vi "target_old.vi"() -> ()   [LabVIEW 2011]
uses:
  Output - Cluster.ctl
  Input - Cluster.ctl
  <vilib>/Platform/TimedLoop/XDataNode/timing_clust.ctl
  <vilib>/Platform/TimedLoop/XDataNode/nitl_modes.ctl
  <vilib>/Platform/TimedLoop/XDataNode/wakeup.ctl
  <vilib>/functionblocks/Counter/Count Up/Count Up.vi
  <vilib>/functionblocks/Control/PID/PID.vi
  <vilib>/Platform/TimedLoop/XDataNode/XDataNode.xnode
  <vilib>/functionblocks/FB Core/FB Core.xnode
  <vilib>/Platform/TimedLoop/XDataNode/XDNodeRunTimeDep.lvlib
  <vilib>/functionblocks/NI_FunctionBlock Libraries.lvlib
panel:
  in  "Output - Cluster":T1 {"DS-3 [bar]" format="%#.2g"; "TS-6 [°C]" format="%#.2g"; "GZ-1 [dl]" format="%.0g"; "TS-5 [°C]" format="%#.2g"; "pHS-1 [pH]" format="%.2g"; "TS-4 [°C]" format="%#.2g"; "FS-2 [l]" format="%.2g"; "FS-1 [l]" format="%.2g"}
  # "The Network Variable Engine and Variable Client Support must be installed on the RT target\nfor this application to function properly. If the Network Variable Engine is not supported on\nthe target (e.g.  FP-2000 with <32MB of RAM), open the project and move the variable library\nto My Computer in the project. Doing this will deploy the variables to localhost but\nwill still require that Variable Client Support be installed on the RT target."
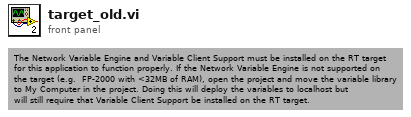
[diagram p1: front panel]
types:
  T1 = typedef "Output - Cluster.ctl" = cluster{"DFS-1 [dl]":u64, "FS-3 [l]":dbl, "DFS-1 [l/min]":dbl, "DS-1 [bar]":dbl, "V-10 ZU":bool, "V-14 ZU":bool, "FS-1 [l]":dbl, "FS-2 [l]":dbl, "TS-4 [°C]":dbl, "HS-1":bool, "V-13 [%]":u8, "V-15 [%]":u8, "P-4 [%]":u8, "P-5 [%]":u8, "Dosierung":bool, "MR Max Füllstand":bool, "MR Min Füllstand":bool, "Dosiermenge [l]":sgl, "V-14 AUF":bool, "V-10 AUF":bool, "T-1 Max Füllstand":bool, "T-1 Min Füllstand":bool, "T-2 Max Füllstand":bool, "T-2 Min Füllstand":bool, "pHS-1 [pH]":dbl, "P-4 RUN":bool, "P-5 RUN ":bool, "V-33 AUF":bool, "V-33 ZU":bool, "V-34 AUF":bool, "V-34 ZU":bool, "P-4 ERR":bool, "P-5 ERR":bool, "TS-5 [°C]":dbl, "GZ-1 [dl]":u64, "TS-6 [°C]":dbl, "DS-3 [bar]":dbl}
  T2 = cluster{"Durchflussregelung":dbl, "Temperaturregelung":bool, "STOP":bool, "Period":i64, "Zirkulation":u64, "Dosierung Zeit":u64}
  T3 = typedef "XDNodeRunTimeDep.lvlib/timing_clust.ctl" = cluster{"Expected End [f-1]":u64, "Actual End [f-1]":u64, "Finished Late? [f-1]":bool, "Expected End [i-1]":u64, "Actual End [i-1]":u64, "Finished Late? [i-1]":bool, "Expected Start [i]":u64, "Actual Start [i]":u64, "Expected Start [f]":u64, "Actual Start [f]":u64, "Source Name":string, "Structure Name":string, "Period":i64, "Deadline":i64, "Offset":i64, "Start":i64, "Priority":i32, "Timeout":i32, "Mode":T4, "Wakeup Reason":T5, "Error":errorcluster, "Source Type":string, "Secondary Source Type":string, "Global End Time":u64, "Global Start Time":u64, "Frame Duration":u64, "Iteration Duration":u64, "Assigned CPU":i32, "I/O Scan Engine Mode":u32}
  T4 = typedef "XDNodeRunTimeDep.lvlib/nitl_modes.ctl" = enum32{"No Change", "Process missed periods, maintain original phase", "Discard missed periods, maintain original phase", "Process missed periods, ignore original phase", "Discard missed periods, ignore original phase"}
  T5 = typedef "XDNodeRunTimeDep.lvlib/wakeup.ctl" = enum32{"Normal", "Aborted", "Asynchronous wakeup", "Timing source error", "Timed loop error", "Timeout"}
  T6 = enum16{"open", "replace", "create", "open or create", "replace or create", "replace or create with confirmation"}
  T7 = typedef "Input - Cluster.ctl" = cluster{"V-13 [%]":u8, "V-15 [%]":u8, "Log-Target":bool, "P-4":bool, "P-4 Drehzahl [%]":u8, "Temperaturregelung":bool, "Überdruckregelung":bool, "Füllstandsregulierung":bool, "V-10":bool, "Log-Host":bool, "V-14":bool, "P-5":bool, "P-5 Drehzahl [%]":u8, "HS-1":bool, "Füllstand  P":sgl, "Füllstand I":sgl, "Füllstand D":sgl, "Füllstand Soll [l]":sgl, "Druck  P":sgl, "Druck I":sgl, "Druck D":sgl, "Druck Soll [bar]":sgl, "Temp Soll [°C]":sgl, "Dosierung":bool, "Dosiermenge [l]":sgl, "Dosiergeschw. [l/min]":sgl, "Tank":bool, "Hysterese [°C]":sgl, "MR Füllstandsüberwachung":bool, "Tank Füllstandsüberwachung":bool, "Log Target [ms]":u32, "Log Host [s]":u32, "P-5 EIN [min]":u8, "P-5 AUS [min]":u8, "Zirkulation":bool, "V-33":bool, "V-34":bool}
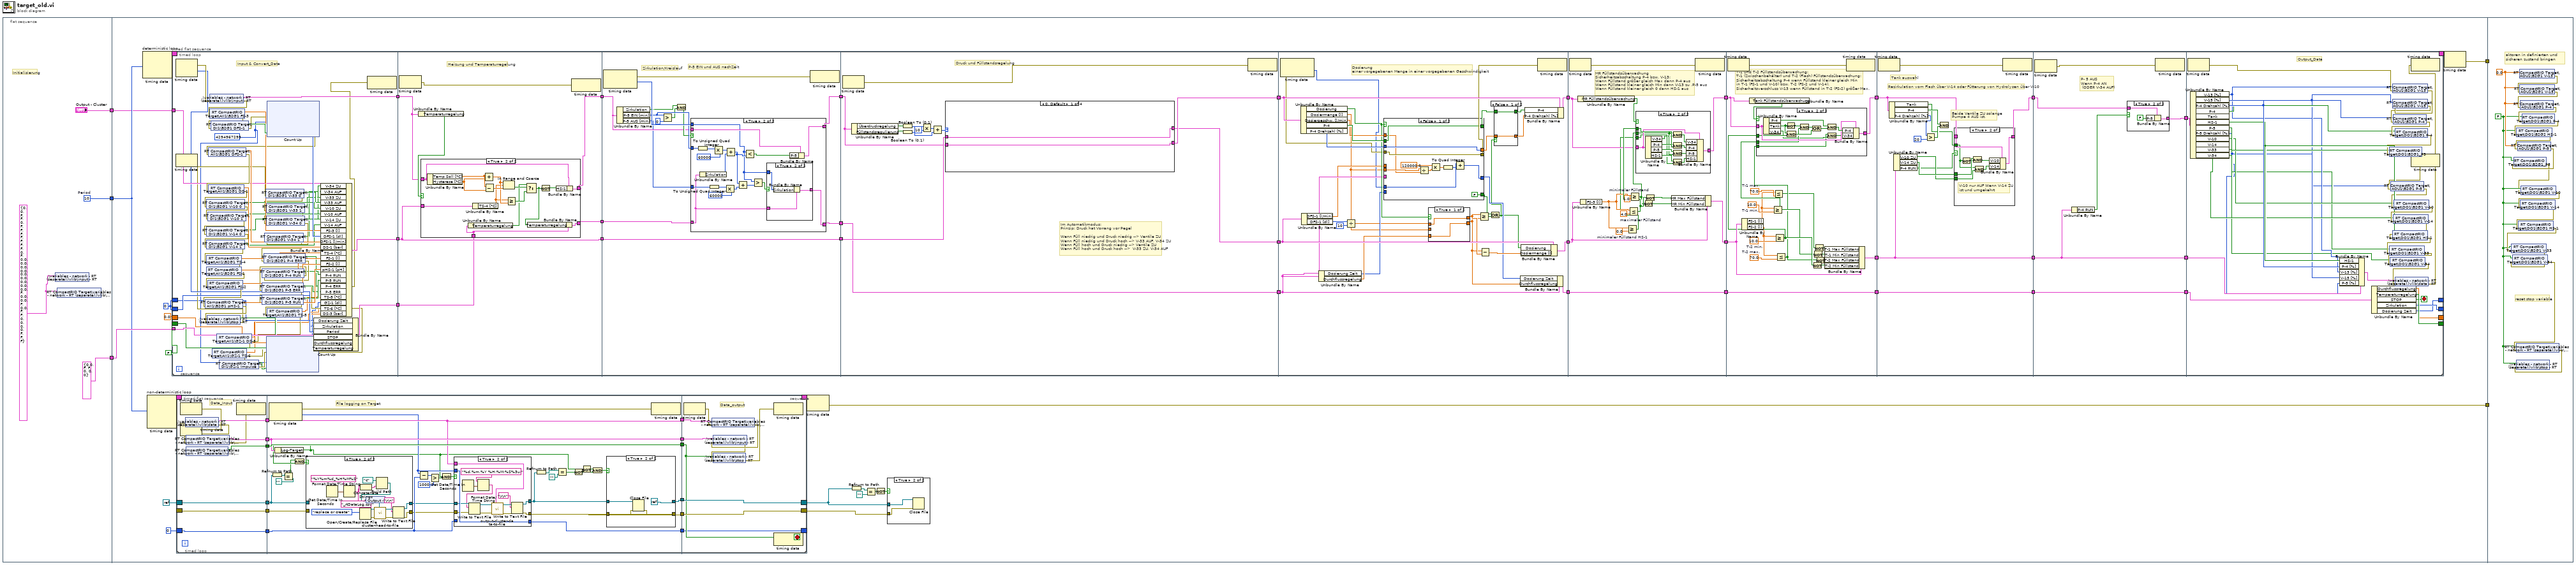
[diagram p0: block diagram]
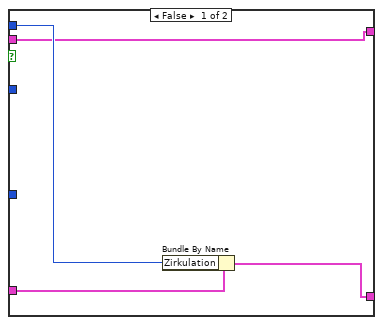
[diagram p7: hidden frame]
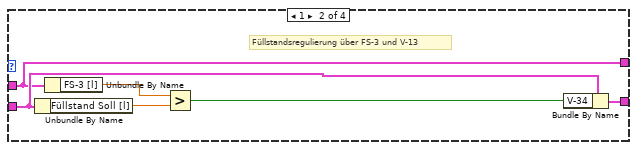
[diagram p9: hidden frame]
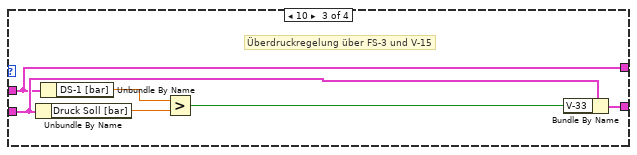
[diagram p10: hidden frame]
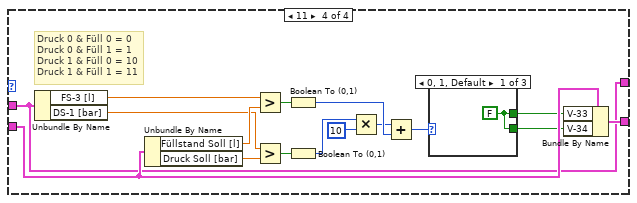
[diagram p11: hidden frame]
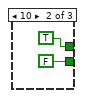
[diagram p12: hidden frame]
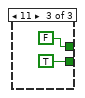
[diagram p13: hidden frame]
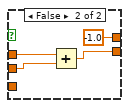
[diagram p14: hidden frame]
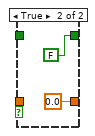
[diagram p15: hidden frame]
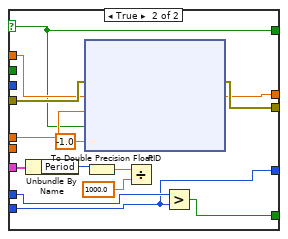
[diagram p16: hidden frame]
diagram:
  n1 = flat-sequence {
    tunnel: [T2 {"Durchflussregelung"=0.0, "Temperaturregelung"=FALSE, "STOP"=FALSE, "Period"=0, "Zirkulation"=0, "Dosierung Zeit"=0} ("rt_vars")] -> w5
    tunnel: [w7] -> w4
    tunnel: ["Output - Cluster"] -> w3
    tunnel: w5 -> [w15]
    tunnel: w4 -> [w14]
    tunnel: w3 -> [w13]
    tunnel: [w12] -> w2
    tunnel: [w11] -> w1
    tunnel: w2 -> [_]
    tunnel: w1 -> [_]
    frame #0 {
      w7 = i64 10  # Period
      w9 = T7 {"V-13 [%]"=0, "V-15 [%]"=0, "Log-Target"=FALSE, "P-4"=FALSE, "P-4 Drehzahl [%]"=0, "Temperaturregelung"=FALSE, "Überdruckregelung"=FALSE, "Füllstandsregulierung"=FALSE, "V-10"=FALSE, "Log-Host"=FALSE, "V-14"=FALSE, "P-5"=FALSE, "P-5 Drehzahl [%]"=0, "HS-1"=FALSE, "Füllstand  P"=0.0, "Füllstand I"=0.0, "Füllstand D"=0.0, "Füllstand Soll [l]"=0.0, "Druck  P"=0.0, "Druck I"=0.0, "Druck D"=0.0, "Druck Soll [bar]"=0.0, "Temp Soll [°C]"=0.0, "Dosierung"=FALSE, "Dosiermenge [l]"=0.0, "Dosiergeschw. [l/min]"=0.0, "Tank"=FALSE, "Hysterese [°C]"=0.0, "MR Füllstandsüberwachung"=FALSE, "Tank Füllstandsüberwachung"=FALSE, "Log Target [ms]"=0, "Log Host [s]"=0, "P-5 EIN [min]"=0, "P-5 AUS [min]"=0, "Zirkulation"=FALSE, "V-33"=FALSE, "V-34"=FALSE} ("Input - Cluster")
      # "Initialisierung"
      n2 = shared-variable ".\\variables - network - RT (separate).lvlib\\input - RT"(w9) -> ()  [unwired: 1 in, 1 out]
      n3 = shared-variable "RT CompactRIO Target\\variables - network - RT (separate).lvlib\\input - network"(w9) -> ()  [unwired: 1 in, 1 out]
    }
    frame #1 {
      w10 = u64 0
      n4 = node-c288 ("Input Node")(w14) -> (w29:T3)  [unwired: 2 in]
      n5 = node-c288 ("Input Node")(w14) -> (w27:T3)  [unwired: 3 in]
      n6 = timed-loop "deterministic loop" {
        timing: w29 -> [_]
        timing-out: [_] -> w28
        shift-right: [w178] -> _
        shift-left: 0.0 -> [w177]
        shift-right: [w176] -> _
        shift-left: FALSE ("Temperaturregelung") -> [w174]
        tunnel: w15 -> [w175]
        tunnel: w13 -> [w173]
        shift-right: [w172] -> _
        shift-left: w10 -> [w171]
        shift-right: [w170] -> _
        shift-left: w10 -> [w169]
        stop <- w781 stop-if-true
        n7 = timed-sequence {
          timing: _ -> [_]
          timing-out: _ -> [_]
          tunnel: [w213] -> w178
          tunnel: w177 -> [w212]
          tunnel: [w209] -> w176
          tunnel: w175 -> [w208]
          tunnel: w174 -> [w206]
          tunnel: w173 -> [w201]
          tunnel: [w188] -> w172
          tunnel: w171 -> [w187]
          tunnel: [w180] -> w170
          tunnel: w169 -> [w179]
          n8 = timed-flat-sequence {
            tunnel: [w281] -> w211
            tunnel: [w276] -> w210
            tunnel: w212 -> [w259]
            tunnel: w208 -> [w258]
            tunnel: [w257] -> w207
            tunnel: w206 -> [w256]
            tunnel: w201 -> [w250]
            tunnel: w187 -> [w241]
            tunnel: w179 -> [w226]
            tunnel: w211 -> [w378]
            tunnel: w210 -> [w382]
            tunnel: [w382] -> w194
            tunnel: w207 -> [w381]
            tunnel: [w380] -> w192
            tunnel: [w377] -> w190
            tunnel: w194 -> [w406]
            tunnel: [w406] -> w193
            tunnel: w192 -> [w417]
            tunnel: [w416] -> w191
            tunnel: w190 -> [w409]
            tunnel: [w408] -> w189
            tunnel: [w463] -> w215
            tunnel: w193 -> [w462]
            tunnel: [w461] -> w214
            tunnel: w191 -> [w453]
            tunnel: [w453] -> w205
            tunnel: w189 -> [w452]
            tunnel: w215 -> [w534]
            tunnel: [w532] -> w200
            tunnel: w214 -> [w533]
            tunnel: [w527] -> w199
            tunnel: w205 -> [w515]
            tunnel: [w519] -> w198
            tunnel: w200 -> [w647]
            tunnel: [w648] -> w204
            tunnel: w199 -> [w656]
            tunnel: [w653] -> w203
            tunnel: w198 -> [w658]
            tunnel: [w658] -> w202
            tunnel: w204 -> [w679]
            tunnel: [w694] -> w197
            tunnel: w203 -> [w693]
            tunnel: [w692] -> w196
            tunnel: w202 -> [w698]
            tunnel: [w698] -> w195
            tunnel: w197 -> [w730]
            tunnel: [w729] -> w186
            tunnel: w196 -> [w722]
            tunnel: [w722] -> w184
            tunnel: w195 -> [w731]
            tunnel: [w731] -> w182
            tunnel: w186 -> [w749]
            tunnel: [w748] -> w185
            tunnel: w184 -> [w747]
            tunnel: [w747] -> w183
            tunnel: w182 -> [w751]
            tunnel: [w751] -> w181
            tunnel: w185 -> [w789]
            tunnel: w183 -> [w787]
            tunnel: [w782] -> w213
            tunnel: [w783] -> w209
            tunnel: w181 -> [w784]
            tunnel: [w765] -> w188
            tunnel: [w761] -> w180
            frame #0 {
              w219 = u32 4294967295 ("preset value")
              # "Input & Convert_Data"
              n9 = node-c288 ("Output Node")() -> (w280:errorcluster, w247:i64)  [unwired: 1 in]
              n10 = shared-variable ".\\variables - network - RT (separate).lvlib\\input - RT"(error in=w280) -> (w281:T7, error out=w274:errorcluster)
              n11 = shared-variable "RT CompactRIO Target\\AII1\\B2G1 FS-3"(error in=w274) -> (w275:dbl, error out=w273:errorcluster)
              n12 = shared-variable "RT CompactRIO Target\\DI1\\B2G1 DFS-1"(error in=w273) -> (w282:bool, error out=w272:errorcluster)
              n13 = xnode "Count Up"("error in"=w272, "preset value"=w219, "count up"=w282) -> ("error out"=w271:errorcluster, "counter value"=w279:u32)  [unwired: 1 in, 1 out]
              n14 = shared-variable "RT CompactRIO Target\\AII1\\B2G1 DFS-1"(error in=w271) -> (w278:dbl, error out=w270:errorcluster)
              n15 = shared-variable "RT CompactRIO Target\\AII1\\B2G1 DS-1"(error in=w270) -> (w277:dbl, error out=w269:errorcluster)
              n16 = shared-variable "RT CompactRIO Target\\DI1\\B2G1 V-10 0"(error in=w269) -> (w265:bool, error out=w268:errorcluster)
              n17 = shared-variable "RT CompactRIO Target\\DI1\\B2G1 V-10 1"(error in=w268) -> (w264:bool, error out=w267:errorcluster)
              n18 = shared-variable "RT CompactRIO Target\\DI1\\B2G1 V-14 0"(error in=w267) -> (w263:bool, error out=w266:errorcluster)
              n19 = shared-variable "RT CompactRIO Target\\DI1\\B2G1 V-14 1"(error in=w266) -> (w262:bool, error out=w261:errorcluster)
              n20 = shared-variable "RT CompactRIO Target\\AII1\\B2G1 TS-4"(error in=w261) -> (w260:dbl, error out=w252:errorcluster)
              n21 = shared-variable "RT CompactRIO Target\\AII1\\B2G1 FS-1"(error in=w252) -> (w254:dbl, error out=w251:errorcluster)
              n22 = shared-variable "RT CompactRIO Target\\AII1\\B2G1 FS-2"(error in=w251) -> (w253:dbl, error out=w249:errorcluster)
              n23 = shared-variable "RT CompactRIO Target\\AII1\\B2G1 pHS-1"(error in=w249) -> (w248:dbl, error out=w233:errorcluster)
              n24 = shared-variable ".\\variables - network - RT (separate).lvlib\\stop - RT"(error in=w233) -> (w255:bool, error out=w232:errorcluster)
              n25 = shared-variable "RT CompactRIO Target\\DI1\\B2G1 V-33 0"(error in=w232) -> (w245:bool, error out=w246:errorcluster)
              n26 = shared-variable "RT CompactRIO Target\\DI1\\B2G1 V-33 1"(error in=w246) -> (w244:bool, error out=w243:errorcluster)
              n27 = shared-variable "RT CompactRIO Target\\DI1\\B2G1 V-34 0"(error in=w243) -> (w240:bool, error out=w242:errorcluster)
              n28 = shared-variable "RT CompactRIO Target\\DI1\\B2G1 V-34 1"(error in=w242) -> (w239:bool, error out=w238:errorcluster)
              n29 = shared-variable "RT CompactRIO Target\\DI1\\B2G1 P-4 ERR"(error in=w238) -> (w229:bool, error out=w237:errorcluster)
              n30 = shared-variable "RT CompactRIO Target\\DI1\\B2G1 P-4 RUN"(error in=w237) -> (w231:bool, error out=w236:errorcluster)
              n31 = shared-variable "RT CompactRIO Target\\DI1\\B2G1 P-5 ERR"(error in=w236) -> (w228:bool, error out=w235:errorcluster)
              n32 = shared-variable "RT CompactRIO Target\\DI1\\B2G1 P-5 RUN"(error in=w235) -> (w230:bool, error out=w234:errorcluster)
              n33 = shared-variable "RT CompactRIO Target\\AII1\\B2G1 TS-5"(error in=w234) -> (w227:dbl, error out=w225:errorcluster)
              n34 = shared-variable "RT CompactRIO Target\\AII1\\GZ-1 DS-3"(error in=w225) -> (w217:dbl, error out=w224:errorcluster)
              n35 = shared-variable "RT CompactRIO Target\\AII1\\GZ-1 TS-6"(error in=w224) -> (w218:dbl, error out=w223:errorcluster)
              n36 = shared-variable "RT CompactRIO Target\\DI1\\GZ-1 Impulse"(error in=w223) -> (w220:bool, error out=w221:errorcluster)
              n37 = xnode "Count Up"("error in"=w221, "preset value"=w219, "count up"=w220) -> ("error out"=w222:errorcluster, "counter value"=w216:u32)  [unwired: 1 in, 1 out]
              n38 = Bundle By Name(cluster=w258, "Dosierung Zeit"=w226, "Zirkulation"=w241, "Period"=w247, "STOP"=w255, "Durchflussregelung"=w259, "Temperaturregelung"=w256) -> (w257:T2)
              n39 = Bundle By Name(cluster=w250, "V-34 ZU"=w240, "V-34 AUF"=w239, "V-33 ZU"=w244, "V-33 AUF"=w245, "V-10 ZU"=w265, "V-10 AUF"=w264, "V-14 ZU"=w263, "V-14 AUF"=w262, "FS-3 [l]"=w275, "DFS-1 [dl]"=w279, "DFS-1 [l/min]"=w278, "DS-1 [bar]"=w277, "TS-4 [°C]"=w260, "FS-1 [l]"=w254, "FS-2 [l]"=w253, "pHS-1 [pH]"=w248, "P-4 RUN"=w231, "P-5 RUN"=w230, "P-4 ERR"=w229, "P-5 ERR"=w228, "TS-5 [°C]"=w227, "GZ-1 [dl]"=w216, "TS-6 [°C]"=w218, "DS-3 [bar]"=w217) -> (w276:T1)
              n40 = node-c288 ("Input Node")(w222) -> ()  [unwired: 1 out]
            }
            frame #1 {
              # "Heizung und Temperaturregelung"
              n41 = node-c288() -> (w383:errorcluster)  [unwired: 1 in]
              n42 = Unbundle By Name(w378) -> ("Temperaturregelung"=w379:bool)
              n43 = case shown="True" w379 {
                tunnel: w382 -> [_ w395]
                tunnel: w381 -> [w385 w392]
                tunnel: [w385 w390] -> w380
                tunnel: w378 -> [w384 w386]
                tunnel: [w384 w388] -> w377
                frame False {
                }
                frame True {
                  n44 = Unbundle By Name(w386) -> ("Temp Soll [°C]"=w396:sgl, "Hysterese [°C]"=w389:sgl)
                  n45 = Unbundle By Name(w392) -> ("Temperaturregelung"=w393:bool)
                  n46 = Unbundle By Name(w395) -> ("TS-4 [°C]"=w394:dbl)
                  n47 = Add(x=w396, y=w389) -> (x+y=w398:sgl)
                  n48 = Subtract(x=w396, y=w389) -> (x-y=w400:sgl)
                  n49 = In Range and Coerce(upper limit=w398, x=w394, lower limit=w400) -> (In Range?=w399:bool)  [unwired: 1 out]
                  n50 = Greater Or Equal?(x=w394, y=w398) -> (x >= y?=w397:bool)
                  n51 = Select(t=w393, s=w399, f=w397) -> (s? t:f=w391:bool)
                  n52 = Bundle By Name(cluster=w392, "Temperaturregelung"=w391) -> (w390:T2)
                  n53 = Not(x=w391) -> (.not. x?=w387:bool)
                  n54 = Bundle By Name(cluster=w386, "HS-1"=w387) -> (w388:T7)
                }
              }
              n55 = node-c288(w383) -> ()  [unwired: 1 out]
            }
            frame #2 {
              # "P-5 EIN und AUS nachZeit"
              # "Zirkulation/Kreislauf"
              n56 = node-c288() -> (w418:errorcluster, w415:i64)  [unwired: 1 in]
              n57 = Unbundle By Name(w409) -> ("Zirkulation"=w410:bool, "P-5 EIN [min]"=w413:u8, "P-5 AUS [min]"=w407:u8)
              n58 = Greater?(x=w413, y=u8 0) -> (0:w412:bool)
              n59 = And(x=w410, y=w412) -> (x .and. y?=w411:bool)
              n60 = case shown="True" w411 {
                tunnel: w417 -> [w422 w425]
                tunnel: [w421 w424] -> w416
                tunnel: w415 -> [w420 w423]
                tunnel: w413 -> [_ w436]
                tunnel: w409 -> [w419 w435]
                tunnel: [w419 w431] -> w408
                tunnel: w407 -> [_ w430]
                frame False {
                  n61 = Bundle By Name(cluster=w422, "Zirkulation"=w420) -> (w421:T2)
                }
                frame True {
                  n62 = To Unsigned Quad Integer(1:w436) -> (0:w437:u64)
                  n63 = Unbundle By Name(w425) -> ("Zirkulation"=w440:u64)
                  n64 = To Unsigned Quad Integer(1:w430) -> (0:w432:u64)
                  n65 = Multiply(x=w437, y=u64 60000) -> (x*y=w439:u64)
                  n66 = Multiply(x=w432, y=u64 60000) -> (x*y=w429:u64)
                  n67 = Add(x=w439, y=w440) -> (x+y=w428:u64)
                  n68 = Add(x=w428, y=w429) -> (x+y=w427:u64)
                  n69 = Less?(x=w423, y=w428) -> (x < y?=w434:bool)
                  n70 = Greater?(x=w423, y=w427) -> (0:w426:bool)
                  n71 = case shown="True" w426 {
                    tunnel: w425 -> [w441 w444]
                    tunnel: [w441 w443] -> w424
                    tunnel: w423 -> [_ w442]
                    frame False {
                    }
                    frame True {
                      n72 = Bundle By Name(cluster=w444, "Zirkulation"=w442) -> (w443:T2)
                    }
                  }
                  n73 = Bundle By Name(cluster=w435, "P-5"=w434) -> (w431:T7)
                }
              }
              n74 = node-c288(w418) -> ()  [unwired: 1 out]
            }
            frame #3 {
              # "Im Automatikmodus:\nPrinzip: Druck hat Vorrang vor Pegel\n\nWenn Füll niedrig und Druck niedrig --> Ventile ZU\nWenn Füll niedrig und Druck hoch --> V-33 AUF, V-34 ZU\nWenn Füll hoch und Druck niedrig --> Ventile ZU\nWenn Füll hoch und Druck hoch -->  V-33 ZU, V-34 AUF"
              # "Druck und Füllstandsregelung"
              n75 = node-c288() -> (w451:errorcluster)  [unwired: 1 in]
              n76 = Unbundle By Name(w452) -> ("Überdruckregelung"=w460:bool, "Füllstandsregulierung"=w459:bool)
              n77 = Boolean To (0,1)(Boolean=w459) -> (0, 1=w455:i16)
              n78 = Boolean To (0,1)(Boolean=w460) -> (0, 1=w458:i16)
              n79 = Multiply(x=w458, y=i16 10) -> (x*y=w456:i16)
              n80 = Add(x=w456, y=w455) -> (x+y=w454:i16)
              n81 = case shown="0, Default" w454 {
                tunnel: w452 -> [w465 w471 w477 w481]
                tunnel: [w465 w470 w476 w482] -> w463
                tunnel: w462 -> [w464 w469 w475 w480]
                tunnel: [w464 w469 w475 w480] -> w461
                frame 0, Default {
                }
                frame 1 {
                  # "Füllstandsregulierung über FS-3 und V-13"
                  n82 = Unbundle By Name(w471) -> ("Füllstand Soll [l]"=w468:sgl)
                  n83 = Unbundle By Name(w469) -> ("FS-3 [l]"=w467:dbl)
                  n84 = Greater?(x=w467, y=w468) -> (0:w466:bool)
                  n85 = Bundle By Name(cluster=w471, "V-34"=w466) -> (w470:T7)
                }
                frame 10 {
                  # "Überdruckregelung über FS-3 und V-15"
                  n86 = Unbundle By Name(w477) -> ("Druck Soll [bar]"=w473:sgl)
                  n87 = Unbundle By Name(w475) -> ("DS-1 [bar]"=w474:dbl)
                  n88 = Greater?(x=w474, y=w473) -> (0:w472:bool)
                  n89 = Bundle By Name(cluster=w477, "V-33"=w472) -> (w476:T7)
                }
                frame 11 {
                  # "Druck 0 & Füll 0 = 0\nDruck 0 & Füll 1 = 1\nDruck 1 & Füll 0 = 10\nDruck 1 & Füll 1 = 11"
                  n90 = Unbundle By Name(w480) -> ("FS-3 [l]"=w492:dbl, "DS-1 [bar]"=w486:dbl)
                  n91 = Unbundle By Name(w481) -> ("Füllstand Soll [l]"=w493:sgl, "Druck Soll [bar]"=w487:sgl)
                  n92 = Greater?(x=w492, y=w493) -> (0:w490:bool)
                  n93 = Greater?(x=w486, y=w487) -> (0:w491:bool)
                  n94 = Boolean To (0,1)(Boolean=w490) -> (0, 1=w489:i16)
                  n95 = Boolean To (0,1)(Boolean=w491) -> (0, 1=w485:i16)
                  n96 = Multiply(x=w485, y=i16 10) -> (x*y=w483:i16)
                  n97 = Add(x=w483, y=w489) -> (x+y=w488:i16)
                  n98 = case shown="0, 1, Default" w488 {
                    tunnel: [w494 TRUE ("auto? (T)") FALSE ("auto? (T)")] -> w479
                    tunnel: [w494 FALSE ("auto? (T)") TRUE ("auto? (T)")] -> w478
                    frame 0, 1, Default {
                      w494 = FALSE ("auto? (T)")
                    }
                    frame 10 {
                    }
                    frame 11 {
                    }
                  }
                  n99 = Bundle By Name(cluster=w481, "V-33"=w479, "V-34"=w478) -> (w482:T7)
                }
              }
              n100 = node-c288(w451) -> ()  [unwired: 1 out]
            }
            frame #4 {
              # "Dosierung \neiner vorgegebenen Menge in einer vorgegebenen Geschwindigkeit"
              n101 = node-c288() -> (w516:errorcluster, w509:i64)  [unwired: 1 in]
              n102 = Unbundle By Name(w534) -> ("Dosierung"=w523:bool, "Dosiermenge [l]"=w504:sgl, "Dosiergeschw. [l/min]"=w528:sgl, "P-4"=w531:bool, "P-4 Drehzahl [%]"=w530:u8)
              n103 = Unbundle By Name(w533) -> ("DFS-1 [l/min]"=w511:dbl, "DFS-1 [dl]"=w512:u64)
              n104 = Unbundle By Name(w515) -> ("Dosierung Zeit"=w510:u64, "Durchflussregelung"=w517:dbl)
              n105 = Divide(x=w512, y=u64 10) -> (x/y=w505:dbl)
              n106 = case shown="False" w523 {
                selector: w523 -> [_ w565]
                tunnel: [w556 w565] -> w514
                tunnel: w531 -> [w556 _]
                tunnel: [w555 w568] -> w524
                tunnel: w530 -> [w555 _]
                tunnel: [w554 w570] -> w529
                tunnel: w516 -> [w554 w569]
                tunnel: w528 -> [w545 w567]
                tunnel: w511 -> [_ w566]
                tunnel: w515 -> [_ w561]
                tunnel: w510 -> [_ w558]
                tunnel: w509 -> [w553 w560]
                tunnel: [w552 w558] -> w508
                tunnel: [FALSE w559] -> w506
                tunnel: w504 -> [w546 _]
                frame False {
                  n107 = Divide(x=w546, y=w545) -> (x/y=w549:sgl)
                  n108 = Multiply(x=120000.0, y=w549) -> (x*y=w550:dbl)
                  n109 = To Quad Integer(1:w550) -> (0:w547:i64)
                  n110 = Add(x=w553, y=w547) -> (x+y=w552:i64)
                }
                frame True {
                  n111 = Unbundle By Name(w561) -> ("Period"=w562:i64)
                  n112 = xnode "PID"("error in"=w569, "setpoint"=w567, "process variable"=w566, "auto? (T)"=w565, "dt (s)"=-1.0) -> ("error out"=w570:errorcluster, "output"=w568:dbl)
                  n113 = To Double Precision Float(number=w562) -> (double precision float=w564:dbl)
                  n114 = Divide(x=w564, y=1000.0) -> ()  [unwired: 1 out]
                  n115 = Greater?(x=w560, y=w558) -> (0:w559:bool)
                }
              }
              n116 = case shown="True" w523 {
                tunnel: w504 -> [_ w539]
                tunnel: w505 -> [w535 w538]
                tunnel: [w536 w540] -> w518
                tunnel: w517 -> [w536 _]
                tunnel: [w535 -1.0] -> w520
                frame True {
                }
                frame False {
                  n117 = Add(x=w538, y=w539) -> (x+y=w540:dbl)
                }
              }
              n118 = Greater Or Equal?(x=w520, y=w518) -> (x >= y?=w526:bool)
              n119 = Subtract(x=w518, y=w520) -> (x-y=w521:dbl)
              n120 = Or(x=w506, y=w526) -> (x .or. y?=w507:bool)
              n121 = case shown="False" w507 {
                tunnel: [w542 0.0 ("output")] -> w525
                tunnel: w524 -> [w542 _]
                tunnel: [w541 FALSE ("P-4")] -> w513
                tunnel: w514 -> [w541 _]
                frame False {
                }
                frame True {
                }
              }
              n122 = Bundle By Name(cluster=w515, "Dosierung Zeit"=w508, "Durchflussregelung"=w518) -> (w519:T2)
              n123 = Bundle By Name(cluster=w533, "Dosierung"=w507, "Dosiermenge [l]"=w521) -> (w527:T1)
              n124 = Bundle By Name(cluster=w534, "P-4"=w513, "P-4 Drehzahl [%]"=w525) -> (w532:T7)
              n125 = node-c288(w529) -> ()  [unwired: 1 out]
            }
            frame #5 {
              w644 = 0.0  # minimaler Füllstand HS-1
              w654 = 1.0  # minimaler Füllstand
              w655 = 4.0  # maximaler Füllstand
              # "MR Füllstandsüberwachung\nSicherheitsabschaltung P-4 bzw. V-13:\nWenn Füllstand größer gleich Max dann P-4 aus\nWenn Füllstand kleiner gleich Min dann V-13 zu ,P-5 aus\nWenn Füllstand kleiner gleich 0 dann HS-1 aus"
              n126 = node-c288() -> (w657:errorcluster)  [unwired: 1 in]
              n127 = Unbundle By Name(w647) -> ("MR Füllstandsüberwachung"=w646:bool)
              n128 = Unbundle By Name(w656) -> ("FS-3 [l]"=w645:dbl)
              n129 = Greater Or Equal?(x=w645, y=w644) -> (x >= y?=w643:bool)
              n130 = Less Or Equal?(x=w645, y=w655) -> (x <= y?=w652:bool)
              n131 = Greater Or Equal?(x=w645, y=w654) -> (x >= y?=w650:bool)
              n132 = case shown="True" w646 {
                tunnel: w652 -> [_ w672]
                tunnel: w650 -> [_ w662]
                tunnel: w647 -> [w659 w669]
                tunnel: [w659 w668] -> w648
                tunnel: w643 -> [_ w663]
                frame False {
                }
                frame True {
                  n133 = Unbundle By Name(w669) -> ("V-34"=w661:bool, "P-4"=w671:bool, "P-5"=w667:bool, "HS-1"=w665:bool)
                  n134 = And(x=w662, y=w661) -> (x .and. y?=w660:bool)
                  n135 = And(x=w671, y=w672) -> (x .and. y?=w670:bool)
                  n136 = And(x=w667, y=w662) -> (x .and. y?=w666:bool)
                  n137 = And(x=w665, y=w663) -> (x .and. y?=w664:bool)
                  n138 = Bundle By Name(cluster=w669, "V-34"=w660, "P-4"=w670, "P-5"=w666, "HS-1"=w664) -> (w668:T7)
                }
              }
              n139 = Not(x=w650) -> (.not. x?=w649:bool)
              n140 = Not(x=w652) -> (.not. x?=w651:bool)
              n141 = Bundle By Name(cluster=w656, "MR Max Füllstand"=w651, "MR Min Füllstand"=w649) -> (w653:T1)
              n142 = node-c288(w657) -> ()  [unwired: 1 out]
            }
            frame #6 {
              w683 = 70.0  # T-1 max.
              w686 = 70.0  # T-2 max.
              w695 = 10.0  # T-2 min.
              w696 = 10.0  # T-1 min.
              # "T-1 und T-2 Füllstandsüberwachung:\nT-1 (Zwischenbehälter) und T-2 (Flash) Füllstandsüberwachung:\nSicherheitsabschaltung P-4 wenn Füllstand kleiner gleich Min\nin T-1 (FS-1 und V-10) bzw. T-2 (FS-2 und V-14).\nSicherheitsverschluss V-13 wenn Füllstand in T-2 (FS-2) größer Max."
              n143 = node-c288() -> (w697:errorcluster)  [unwired: 1 in]
              n144 = Unbundle By Name(w693) -> ("FS-1 [l]"=w682:dbl, "FS-2 [l]"=w687:dbl)
              n145 = Unbundle By Name(w679) -> ("Tank Füllstandsüberwachung"=w678:bool)
              n146 = Greater Or Equal?(x=w682, y=w696) -> (x >= y?=w690:bool)
              n147 = Less Or Equal?(x=w682, y=w683) -> (x <= y?=w681:bool)
              n148 = Greater Or Equal?(x=w687, y=w695) -> (x >= y?=w691:bool)
              n149 = Less Or Equal?(x=w687, y=w686) -> (x <= y?=w684:bool)
              n150 = case shown="True" w678 {
                tunnel: w679 -> [w699 w707]
                tunnel: [w699 w706] -> w694
                tunnel: w691 -> [_ w705]
                tunnel: w690 -> [_ w704]
                tunnel: w684 -> [_ w700]
                frame False {
                }
                frame True {
                  n151 = Unbundle By Name(w707) -> ("P-4"=w709:bool, "Tank"=w712:bool, "V-34"=w703:bool)
                  n152 = Not(x=w712) -> (.not. x?=w713:bool)
                  n153 = And(x=w712, y=w705) -> (x .and. y?=w711:bool)
                  n154 = And(x=w713, y=w704) -> (x .and. y?=w701:bool)
                  n155 = Or(x=w701, y=w711) -> (x .or. y?=w710:bool)
                  n156 = And(x=w709, y=w710) -> (x .and. y?=w708:bool)
                  n157 = And(x=w700, y=w703) -> (x .and. y?=w702:bool)
                  n158 = Bundle By Name(cluster=w707, "P-4"=w708, "V-34"=w702) -> (w706:T7)
                }
              }
              n159 = Not(x=w691) -> (.not. x?=w688:bool)
              n160 = Not(x=w690) -> (.not. x?=w689:bool)
              n161 = Not(x=w681) -> (.not. x?=w680:bool)
              n162 = Not(x=w684) -> (.not. x?=w685:bool)
              n163 = Bundle By Name(cluster=w693, "T-1 Max Füllstand"=w680, "T-1 Min Füllstand"=w689, "T-2 Max Füllstand"=w685, "T-2 Min Füllstand"=w688) -> (w692:T1)
              n164 = node-c288(w697) -> ()  [unwired: 1 out]
            }
            frame #7 {
              # "Beide Ventile ZU solange \nPumpe 4 AUS ist."
              # "Rezirkulation vom Flash über V-14 oder Fütterung von Hydrolysen über V-10"
              # "Tank auswahl"
              n165 = node-c288() -> (w723:errorcluster)  [unwired: 1 in]
              n166 = Unbundle By Name(w730) -> ("Tank"=w724:bool, "P-4"=w728:bool, "P-4 Drehzahl [%]"=w727:u8)
              n167 = Unbundle By Name(w722) -> ("V-10 ZU"=w720:bool, "V-14 ZU"=w721:bool, "P-4 RUN"=w719:bool)
              n168 = Greater?(x=w727, y=u8 20) -> (0:w725:bool)
              n169 = And(x=w728, y=w725) -> ()  [unwired: 1 out]
              n170 = case shown="True" w719 {
                tunnel: w730 -> [w732 w740]
                tunnel: [w732 w739] -> w729
                tunnel: w724 -> [_ w734]
                tunnel: w721 -> [_ w737]
                tunnel: w720 -> [_ w733]
                frame False {
                }
                frame True {
                  # "V-10 nur AUF Wenn V-14 ZU\nist und umgekehrt"
                  n171 = Not(x=w734) -> (.not. x?=w736:bool)
                  n172 = And(x=w737, y=w736) -> (x .and. y?=w738:bool)
                  n173 = And(x=w734, y=w733) -> (x .and. y?=w735:bool)
                  n174 = Bundle By Name(cluster=w740, "V-10"=w738, "V-14"=w735) -> (w739:T7)
                }
              }
              n175 = node-c288(w723) -> ()  [unwired: 1 out]
            }
            frame #8 {
              # "P- 5 AUS \nWenn P-4 AN\n (ODER V-34 AUF)"
              n176 = node-c288() -> (w750:errorcluster)  [unwired: 1 in]
              n177 = Unbundle By Name(w747) -> ("P-4 RUN"=w746:bool)
              n178 = case shown="True" w746 {
                tunnel: w749 -> [w752 w755]
                tunnel: [w752 w754] -> w748
                frame False {
                }
                frame True {
                  n179 = Bundle By Name(cluster=w755, "P-5"=FALSE) -> (w754:T7)
                }
              }
              n180 = node-c288(w750) -> ()  [unwired: 1 out]
            }
            frame #9 {
              # "Output_Data"
              n181 = node-c288() -> (w788:errorcluster)  [unwired: 1 in]
              n182 = Unbundle By Name(w789) -> ("V-13 [%]"=w768:u8, "V-15 [%]"=w771:u8, "P-4 Drehzahl [%]"=w779:u8, "P-4"=w774:bool, "HS-1"=w778:bool, "P-5"=w773:bool, "P-5 Drehzahl [%]"=w762:u8, "V-10"=w770:bool, "V-14"=w769:bool, "V-33"=w764:bool, "V-34"=w763:bool)  [unwired: 1 out]
              n183 = Bundle By Name(cluster=w787, "HS-1"=w778, "P-4 [%]"=w779, "V-13 [%]"=w768, "V-15 [%]"=w771, "P-5 [%]"=w762) -> (w786:T1)
              n184 = Unbundle By Name(w784) -> ("Durchflussregelung"=w782:dbl, "Temperaturregelung"=w783:bool, "STOP"=w781:bool, "Zirkulation"=w765:u64, "Dosierung Zeit"=w761:u64)
              n185 = shared-variable "RT CompactRIO Target\\AOU1\\B2G1 V-13"(w768, error in=w788) -> (error out=w793:errorcluster)
              n186 = shared-variable "RT CompactRIO Target\\AOU1\\B2G1 V-15"(w771, error in=w793) -> (error out=w792:errorcluster)
              n187 = shared-variable "RT CompactRIO Target\\AOU1\\B2G1 P-4"(w779, error in=w792) -> (error out=w791:errorcluster)
              n188 = shared-variable "RT CompactRIO Target\\DO1\\B2G1 P-4"(w774, error in=w791) -> (error out=w777:errorcluster)
              n189 = shared-variable "RT CompactRIO Target\\DO1\\B2G1_P5"(w773, error in=w777) -> (error out=w776:errorcluster)
              n190 = shared-variable "RT CompactRIO Target\\AOU1\\B2G1 P-5"(w762, error in=w776) -> (error out=w775:errorcluster)
              n191 = shared-variable "RT CompactRIO Target\\DO1\\B2G1 V-10"(w770, error in=w775) -> (error out=w785:errorcluster)
              n192 = shared-variable "RT CompactRIO Target\\DO1\\B2G1 V-14"(w769, error in=w785) -> (error out=w780:errorcluster)
              n193 = shared-variable "RT CompactRIO Target\\DO1\\B2G1 HS-1"(w778, error in=w780) -> (error out=w772:errorcluster)
              n194 = shared-variable "RT CompactRIO Target\\DO1\\B2G1 V-33"(w764, error in=w772) -> (error out=w767:errorcluster)
              n195 = shared-variable "RT CompactRIO Target\\DO1\\B2G1 V-34"(w763, error in=w767) -> (error out=w766:errorcluster)
              n196 = shared-variable ".\\variables - network - RT (separate).lvlib\\data - RT"(w786, error in=w766) -> (error out=w790:errorcluster)
              n197 = node-c288(w790) -> ()  [unwired: 1 out]
            }
          }
        }
        n198 = node-c288() -> ()  [unwired: 1 in, 1 out]
        n199 = node-c288() -> ()  [unwired: 1 in, 1 out]
      }
      n200 = timed-loop "non-deterministic loop" {
        timing: w27 -> [_]
        timing-out: [_] -> w26
        shift-right: [w37] -> _
        shift-left: 0 -> [w36]
        shift-right: [w35] -> w19
        shift-left: refnum<k0> refnum -> [w34]
        shift-right: [w33] -> w20
        shift-left: _ -> [w32]
        stop <- w154 stop-if-true
        n201 = timed-sequence {
          timing: _ -> [_]
          timing-out: _ -> [_]
          tunnel: [w46] -> w37
          tunnel: w36 -> [w44]
          tunnel: [w43] -> w35
          tunnel: w34 -> [w41]
          tunnel: [w40] -> w33
          tunnel: w32 -> [w38]
          n202 = timed-flat-sequence {
            tunnel: [w63] -> w55
            tunnel: [w64] -> w54
            tunnel: [w62] -> w49
            tunnel: [w58] -> w45
            tunnel: w44 -> [w58]
            tunnel: [w57] -> w42
            tunnel: w41 -> [w57]
            tunnel: [w56] -> w39
            tunnel: w38 -> [w56]
            tunnel: w55 -> [w98]
            tunnel: w54 -> [w96]
            tunnel: [w88] -> w53
            tunnel: [w89] -> w52
            tunnel: [w98] -> w51
            tunnel: [w97] -> w50
            tunnel: w49 -> [w97]
            tunnel: [w96] -> w48
            tunnel: [w79] -> w47
            tunnel: w45 -> [w90]
            tunnel: w42 -> [w73]
            tunnel: w39 -> [w70]
            tunnel: w53 -> [w156]
            tunnel: w52 -> [w155]
            tunnel: w51 -> [w154]
            tunnel: w50 -> [w153]
            tunnel: w48 -> [w152]
            tunnel: w47 -> [w147]
            tunnel: [w147] -> w46
            tunnel: [w155] -> w43
            tunnel: [w156] -> w40
            frame #0 {
              # "Data_Input"
              n203 = node-c288() -> (w61:errorcluster)  [unwired: 1 in]
              n204 = shared-variable ".\\variables - network - RT (separate).lvlib\\data - RT"(error in=w61) -> (w64:T1, error out=w60:errorcluster)
              n205 = shared-variable "RT CompactRIO Target\\variables - network - RT (separate).lvlib\\input - network"(error in=w60) -> (w62:T7, error out=w59:errorcluster)
              n206 = shared-variable "RT CompactRIO Target\\variables - network - RT (separate).lvlib\\stop - network"() -> (w63:bool)  [unwired: 1 in, 1 out]
              n207 = node-c288(w59) -> ()  [unwired: 1 out]
            }
            frame #1 {
              # "File logging on Target"
              n208 = node-c288() -> (w99:errorcluster, w91:i64)  [unwired: 1 in]
              n209 = Refnum to Path(1:w73) -> (0:w75:path)
              n210 = Unbundle By Name(w97) -> ("Log-Target"=w78:bool)
              n211 = Equal?(x=w75, y=path "") -> (x = y?=w71:bool)
              n212 = And(x=w71, y=w78) -> (x .and. y?=w72:bool)
              n213 = case shown="True" w72 {
                tunnel: [w101 w103] -> w77
                tunnel: [w100 w104] -> w76
                tunnel: w73 -> [w101 _]
                tunnel: w70 -> [w100 _]
                frame False {
                }
                frame True {
                  n214 = Get Date/Time In Seconds() -> (seconds since 1Jan1904=w115:timestamp)
                  n215 = Format Date/Time String(time format string (%c)="%Y%m%d_%H%M%S", seconds (now)=w115) -> (date/time string=w114:string)  [unwired: 1 in]
                  n216 = Concatenate Strings(w114, "_rtDataLog.csv" ("name or relative path")) -> (w111:string)
                  n217 = control-ref of="Output - Cluster"() -> (w107:refnum<vi>)
                  n218 = Build Path(base path=path "c:/", name or relative path=w111) -> (appended path=w110:path)
                  n219 = Open/Create/Replace File(file path (use dialog)=w110, operation (0:open)=T6."replace or create") -> (refnum out=w109:refnum<file>, error out=w108:errorcluster)  [unwired: 4 in, 1 out]
                  n220 = call "cluster-head-to-file.vi"("refnum in"=w109, "error in"=w108, "cluster ref"=w107) -> ("refnum out"=w106:refnum<file>, "error out"=w105:errorcluster)  [unwired: 6 in]
                  n221 = Write to Text File(file (use dialog)=w106, text="\r\n", error in=w105) -> (refnum out=w103:refnum<file>, error out=w104:errorcluster)  [unwired: 1 in, 1 out]
                }
              }
              n222 = Subtract(x=w91, y=w90) -> (x-y=w95:i64)
              n223 = Greater?(x=w95, y=i64 1000) -> (0:w93:bool)
              n224 = And(x=w78, y=w93) -> (x .and. y?=w92:bool)
              n225 = case shown="True" w92 {
                tunnel: [w124 w135] -> w85
                tunnel: [w125 w136] -> w87
                tunnel: w96 -> [_ w140]
                tunnel: w91 -> [_ w139]
                tunnel: [w126 w139] -> w79
                tunnel: w90 -> [w126 _]
                tunnel: w77 -> [w124 w133]
                tunnel: w76 -> [w125 w132]
                frame False {
                }
                frame True {
                  n226 = Get Date/Time In Seconds() -> (seconds since 1Jan1904=w128:timestamp)
                  n227 = Format Date/Time String(time format string (%c)="%d.%m.%Y %H:%M:%S%3u;", seconds (now)=w128) -> (date/time string=w127:string)  [unwired: 1 in]
                  n228 = Write to Text File(file (use dialog)=w133, text=w127, error in=w132) -> (refnum out=w130:refnum<file>, error out=w131:errorcluster)  [unwired: 1 in, 1 out]
                  n229 = call "output-cluster-data-to-file.vi"("refnum in"=w130, "error in"=w131, "Output - Cluster"=w140) -> ("refnum out"=w138:refnum<file>, "error out"=w137:errorcluster)  [unwired: 6 in]
                  n230 = Write to Text File(file (use dialog)=w138, text="\r\n", error in=w137) -> (refnum out=w135:refnum<file>, error out=w136:errorcluster)  [unwired: 1 in, 1 out]
                }
              }
              n231 = Refnum to Path(1:w85) -> (0:w84:path)
              n232 = Equal?(x=w84, y=path "") -> (x = y?=w82:bool)
              n233 = Not(x=w82) -> (.not. x?=w80:bool)
              n234 = Not(x=w78) -> (.not. x?=w81:bool)
              n235 = And(x=w81, y=w80) -> (x .and. y?=w86:bool)
              n236 = case shown="True" w86 {
                tunnel: [w119 refnum<k0> refnum] -> w89
                tunnel: w85 -> [w119 w123]
                tunnel: [w118 w121] -> w88
                tunnel: w87 -> [w118 w122]
                frame False {
                }
                frame True {
                  n237 = Close File(refnum=w123, error in=w122) -> (error out=w121:errorcluster)  [unwired: 1 out]
                }
              }
              n238 = node-c288(w99) -> ()  [unwired: 1 out]
            }
            frame #2 {
              # "Data_output"
              n239 = node-c288() -> (w151:errorcluster)  [unwired: 1 in]
              n240 = shared-variable "RT CompactRIO Target\\variables - network - RT (separate).lvlib\\data - network"(w152, error in=w151) -> (error out=w150:errorcluster)
              n241 = shared-variable ".\\variables - network - RT (separate).lvlib\\input - RT"(w153, error in=w150) -> (error out=w149:errorcluster)
              n242 = shared-variable ".\\variables - network - RT (separate).lvlib\\stop - RT"(w154, error in=w149) -> (error out=w148:errorcluster)
              n243 = node-c288(w148) -> ()  [unwired: 1 out]
            }
          }
        }
        n244 = node-c288() -> ()  [unwired: 1 in, 1 out]
        n245 = node-c288() -> ()  [unwired: 1 in, 1 out]
      }
      n246 = node-c288 ("Output Node")(w26) -> (w12:errorcluster)
      n247 = Refnum to Path(1:w19) -> (0:w18:path)
      n248 = Equal?(x=w18, y=path "") -> (x = y?=w22:bool)
      n249 = Not(x=w22) -> (.not. x?=w21:bool)
      n250 = case shown="True" w21 {
        tunnel: w19 -> [_ w31]
        tunnel: w20 -> [_ w30]
        frame False {
        }
        frame True {
          n251 = Close File(refnum=w31, error in=w30) -> ()  [unwired: 2 out]
        }
      }
      n252 = node-c288 ("Output Node")(w28) -> (w11:errorcluster)
    }
    frame #2 {
      w808 = FALSE ("B2G1 P-4")
      w812 = 0.0 ("B2G1 V-13")
      # "aktoren in definierten und sicheren zustand bringen"
      # "reset stop variable"
      n253 = shared-variable "RT CompactRIO Target\\AOU1\\B2G1 V-13"(w812) -> (error out=w816:errorcluster)  [unwired: 1 in]
      n254 = shared-variable "RT CompactRIO Target\\AOU1\\B2G1 V-15"(w812, error in=w816) -> (error out=w820:errorcluster)
      n255 = shared-variable "RT CompactRIO Target\\AOU1\\B2G1 P-4"(w812, error in=w820) -> (error out=w819:errorcluster)
      n256 = shared-variable "RT CompactRIO Target\\DO1\\B2G1 P-4"(w808, error in=w819) -> (error out=w815:errorcluster)
      n257 = shared-variable "RT CompactRIO Target\\DO1\\B2G2 HS-1"(w808, error in=w815) -> (error out=w817:errorcluster)
      n258 = shared-variable "RT CompactRIO Target\\AOU1\\B2G1 P-5"(w812, error in=w817) -> (error out=w807:errorcluster)
      n259 = shared-variable "RT CompactRIO Target\\DO1\\B2G1_P5"(w808, error in=w807) -> (error out=w806:errorcluster)
      n260 = shared-variable "RT CompactRIO Target\\DO1\\B2G1 V-10"(w808, error in=w806) -> (error out=w814:errorcluster)
      n261 = shared-variable "RT CompactRIO Target\\DO1\\B2G1 V-14"(w808, error in=w814) -> (error out=w818:errorcluster)
      n262 = shared-variable "RT CompactRIO Target\\DO1\\B2G1 HS-1"(w808, error in=w818) -> (error out=w810:errorcluster)
      n263 = shared-variable "RT CompactRIO Target\\DO1\\B2G1 V-33"(w808, error in=w810) -> (error out=w811:errorcluster)
      n264 = shared-variable "RT CompactRIO Target\\DO1\\B2G1 V-34"(w808, error in=w811) -> (error out=w809:errorcluster)
      n265 = shared-variable "RT CompactRIO Target\\variables - network - RT (separate).lvlib\\stop - network"(w808, error in=w809) -> (error out=w813:errorcluster)
      n266 = shared-variable ".\\variables - network - RT (separate).lvlib\\stop - RT"(w808, error in=w813) -> ()  [unwired: 1 out]
    }
  }
